vi "pictureExtensionToType.vi"(11 "Picture File Extension":string) -> (3 "PictureType":T1 items=["BMP"=11, "DIB"=7, "EMF"=2, "EPS"=10, "GIF"=8, "JPEG"=5, "PICT"=4, "PNG"=6, "TIFF"=9, "WMF"=3, "WPG"=12])   [LabVIEW 2017, in "LabVIEW NPOI.lvlib" / "MS-Word.lvclass"]
uses:
  MS-Word.lvclass
  Picture Type.ctl
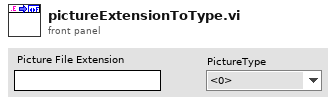
[diagram p1: front panel]
types:
  T1 = typedef "LabVIEW NPOI.lvlib/MS-Word.lvclass/Picture Type.ctl" = i32
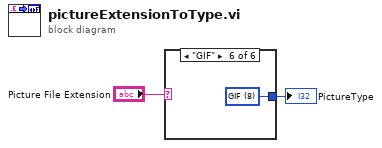
[diagram p0: block diagram]
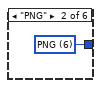
[diagram p3: hidden frame]
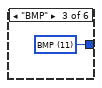
[diagram p4: hidden frame]
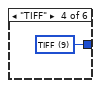
[diagram p5: hidden frame]
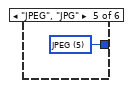
[diagram p6: hidden frame]
diagram:
  n1 = case shown="\"GIF\"" "Picture File Extension" {
    tunnel: [_ w3 w4 w5 w6 w7] -> w1
    frame "False", Default {
    }
    frame "PNG" {
      w3 = T1 6 items=["BMP"=11, "DIB"=7, "EMF"=2, "EPS"=10, "GIF"=8, "JPEG"=5, "PICT"=4, "PNG"=6, "TIFF"=9, "WMF"=3, "WPG"=12] ("PictureType")
    }
    frame "BMP" {
      w4 = T1 11 items=["BMP"=11, "DIB"=7, "EMF"=2, "EPS"=10, "GIF"=8, "JPEG"=5, "PICT"=4, "PNG"=6, "TIFF"=9, "WMF"=3, "WPG"=12] ("PictureType")
    }
    frame "TIFF" {
      w5 = T1 9 items=["BMP"=11, "DIB"=7, "EMF"=2, "EPS"=10, "GIF"=8, "JPEG"=5, "PICT"=4, "PNG"=6, "TIFF"=9, "WMF"=3, "WPG"=12] ("PictureType")
    }
    frame "JPEG", "JPG" {
      w6 = T1 5 items=["BMP"=11, "DIB"=7, "EMF"=2, "EPS"=10, "GIF"=8, "JPEG"=5, "PICT"=4, "PNG"=6, "TIFF"=9, "WMF"=3, "WPG"=12] ("PictureType")
    }
    frame "GIF" {
      w7 = T1 8 items=["BMP"=11, "DIB"=7, "EMF"=2, "EPS"=10, "GIF"=8, "JPEG"=5, "PICT"=4, "PNG"=6, "TIFF"=9, "WMF"=3, "WPG"=12] ("PictureType")
    }
  }
  "PictureType" <- w1
